vi "Get Owning Structure of Terminal.vi"(11 "Terminal":refnum<vi>) -> (2 "Terminal Owned by Structure?":bool, 3 "Owning Structure":refnum<vi>)   [LabVIEW 2017]
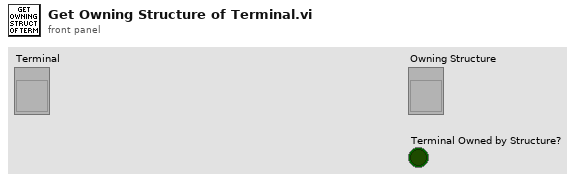
[diagram p1: front panel]
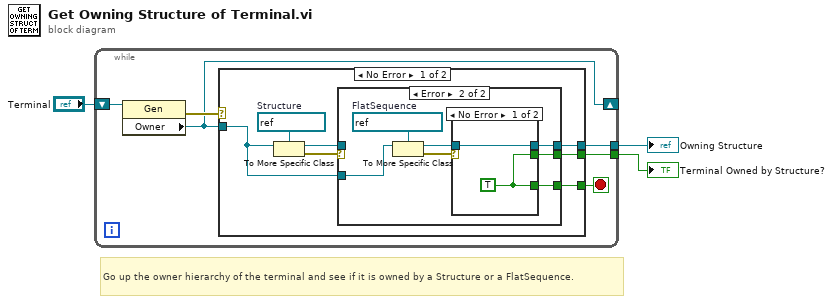
[diagram p0: block diagram]
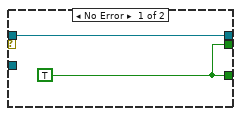
[diagram p2: hidden frame]
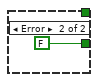
[diagram p3: hidden frame]
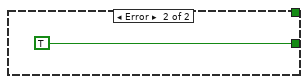
[diagram p4: hidden frame]
diagram:
  # "Go up the owner hierarchy of the terminal and see if it is owned by a Structure or a FlatSequence."
  n1 = while {
    shift-right: [w6] -> _
    shift-left: "Terminal" -> [w9]
    tunnel: [w5] -> w3
    tunnel: [w4] -> w2
    stop <- w8 stop-if-true
    n2 = property class="Gen"(reference=w9) -> (error out=w7:errorcluster, "Owner"=w6:refnum<vi>)  [unwired: 1 in, 1 out]
    n3 = case shown="No Error" w7 {
      tunnel: w6 -> [w10 _]
      tunnel: [w13 TRUE] -> w8
      tunnel: [w12 _] -> w5
      tunnel: [w11 _] -> w4
      frame No Error {
        w16 = refnum<vi> refnum  # Structure
        n4 = To More Specific Class(target class=w16, reference=w10) -> (specific class reference=w14:refnum<vi>, error out=w15:errorcluster)  [unwired: 1 in]
        n5 = case shown="Error" w15 {
          tunnel: w14 -> [w18 _]
          tunnel: [w17 w20] -> w13
          tunnel: [w18 w21] -> w12
          tunnel: [w17 w19] -> w11
          tunnel: w10 -> [_ w24]
          frame No Error {
            w17 = TRUE
          }
          frame Error {
            w25 = refnum<vi> refnum  # FlatSequence
            n6 = To More Specific Class(target class=w25, reference=w24) -> (specific class reference=w22:refnum<vi>, error out=w23:errorcluster)  [unwired: 1 in]
            n7 = case shown="No Error" w23 {
              tunnel: w22 -> [w27 _]
              tunnel: [w27 _] -> w21
              tunnel: [w26 FALSE] -> w20
              tunnel: [w26 _] -> w19
              frame No Error {
                w26 = TRUE
              }
              frame Error {
              }
            }
          }
        }
      }
      frame Error {
      }
    }
  }
  "Owning Structure" <- w3
  "Terminal Owned by Structure?" <- w2
